vi "Dashboard Main.vi"() -> ()   [LabVIEW 2016]
uses:
  <vilib>/Utility/miscctls.llb/LVRowAndColumnTypeDef.ctl
  <vilib>/event_ctls.llb/eventvkey.ctl
  <vilib>/Rock Robotics/Network Tables/NT Read Numeric Array.vi
  <vilib>/Rock Robotics/WPI/Dashboard/WPI_DashboardLogging Global.vi
panel:
  in  "LED Color":T1={"Hue"={107.81818389892578, 139.81818389892578}, "Sat"={176.07142857142858, 255.0}, "Val"={40.53571428571429, 255.0}} {"Hue" scale=0.0..255.0 scale format="%#_3g"}
  in  "Camera Settings Right":T2={"Frame Rate"=30, "Compression"=30, "Size"=1, "DB Camera Config"=FALSE} {"Frame Rate" scale=1.0..30.0; "Compression" scale=100.0..-1.0; "Size" items=["640x480", "320x240", "160x120"]}
  in  "Camera Name Right":string(combo)="No Camera Selection"
  out "Camera Info":cluster{"Mbps LED":bool, "Mbps":dbl, "fps":dbl} {"fps" format="%#.1g"; "Mbps" format="%#.1g"}
  in  "Camera Settings":T2={"Frame Rate"=30, "Compression"=30, "Size"=1, "DB Camera Config"=FALSE} {"Frame Rate" scale=1.0..30.0; "Compression" scale=100.0..-1.0; "Size" items=["640x480", "320x240", "160x120"]}
  in  "TCP":refnum<k5>
  in  "Rec Mode":enum32{"Stop", "Record", "Playback"}(radio)
  out "Robot IP":string
  out "Image Message":string="Timeout in Camera Communications"
  in  "Dashboard Tab":T3(tab)
  in  "Select Auto":string(combo)="Select Autonomous ..."
  out "NT Connection":bool
  out "Mode":T4(ring)=enum."Auto Disabled"
  out "Camera Image Right":T5(plugin-control)
  in  "DB/String 9":string
  in  "DB/String 8":string
  in  "DB/String 7":string
  in  "DB/String 6":string
  in  "DB/String 5":string
  in  "DB/String 4":string
  in  "DB/String 3":string
  in  "DB/String 2":string
  in  "DB/String 1":string
  in  "DB/String 0":string
  in  "DB/Slider 0":dbl(slide) scale=0.0..5.0
  in  "DB/Slider 1":dbl(slide) scale=0.0..5.0
  in  "DB/Slider 2":dbl(slide) scale=0.0..5.0
  in  "DB/Slider 3":dbl(slide) scale=0.0..5.0
  out "DB/LED 3":bool
  out "DB/LED 2":bool
  out "DB/LED 1":bool
  out "DB/LED 0":bool
  in  "DB/Button 3":bool
  in  "DB/Button 2":bool
  in  "DB/Button 1":bool
  in  "DB/Button 0":bool caption="New Name"
  in  "Test Slider":dbl(slide) scale=0.0..100.0 scale format="%#_3g"
  in  "On/Off":bool caption="Solenoid"
  in  "Test Name":u16(ring) items=["Select the test to run..."]
  in  "Test Tree":string(tree)
  in  "Motor":cluster{"Value":dbl, "Enable":bool} {"Value" scale=-1.0..1.0 scale format="%#_3g"}
  out "Progress":T6 {"Test Progress" scale=0.0..100.0}
  in  "Rev/Fwd":cluster{"Forward":bool, "Reverse":bool}
  in  "Test Ring":u16(ring) items=["Monochrome", "Color"]
  out "Cmd Status":string
  in  "Execute Command":bool
  in  "Command Params":string[][](table)
  in  "Command Selection":i32(listbox)
  in  "CheckList":i32(listbox)
  out "Tree":string(tree)
  out "Camera Image":T5(plugin-control)
  out "Background":bool
  in  "Camera Name":string(combo)="No Camera Selection"
  # "HW"
  # "HW"
  # "This tab is a great place for autonomous settings and robot-specific values.\nPlace controls and indicators inside this tab and match name to\nDashboard Variables on robot. You can also delete this comment."
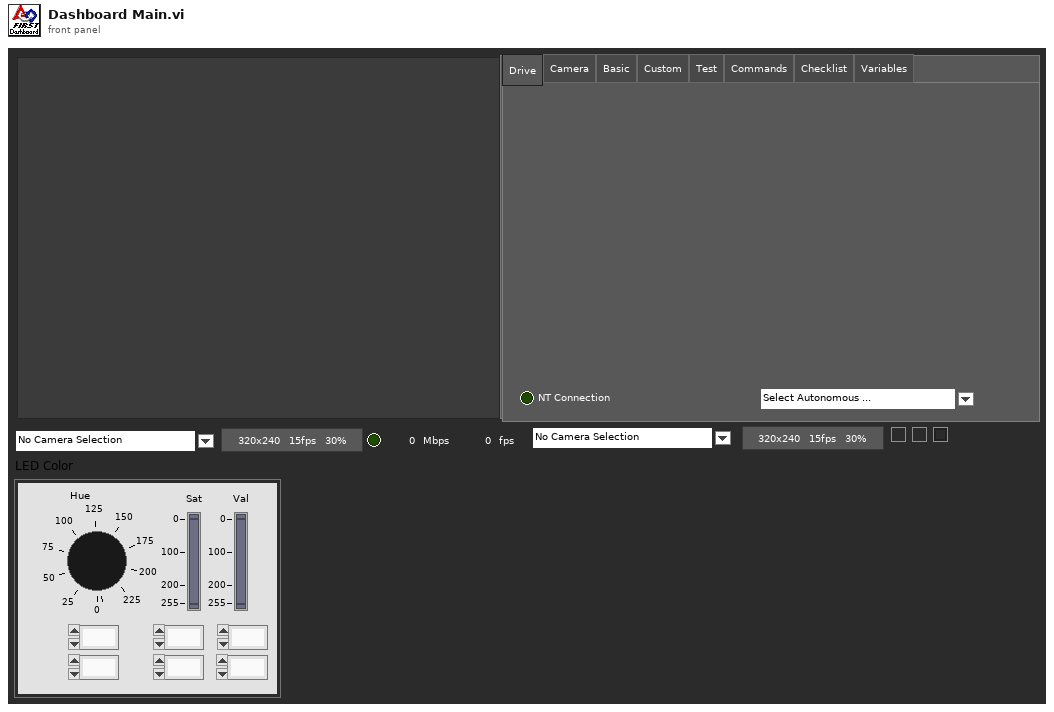
[diagram p1: front panel]
types:
  T1 = cluster{"Hue":cluster{dbl, dbl}, "Sat":cluster{dbl, dbl}, "Val":cluster{dbl, dbl}}
  T2 = cluster{"Frame Rate":i32, "Compression":i32, "Size":u16, "DB Camera Config":bool}
  T3 = enum32{"Drive", "Camera", "Basic", "Custom", "Test", "Commands", "Checklist", "Variables"}
  T4 = enum8{"Tele-Op Disabled", "Tele-Op Enabled", "Auto Disabled", "Auto Enabled", "Test Disabled", "Test Enabled", "Disconnected", "No Code", "E-Stop"}
  T5 = typedef "IMAQ Image.ctl" = refnum<image>
  T6 = cluster{"Test Progress":u8, "Test Progress Text":string}
  T7 = typedef "Image Type" = u32
  T8 = cluster{"IDs":cluster{"RPC field ID":u16, "Unique ID":u16}, "String":string}
  T9 = enum32{"Drive", "Basic", "Custom", "Test", "Checklist", "Variables"}
  T10 = cluster{"Error Strings":string, "Disable Counts":cluster{u16, u16}, "Rail Faults":cluster{u16, u16, u16}, "Robot IP":string, "DB Mode":u8, "Event Info":cluster{"Name":string, "Type":u8, "Number":u16, "Replay":u8}}
  T11 = cluster{"Storage":cluster{"Disk Free":u64, "RAM Block":u32, "RAM free":u32}, "CPU Utilization":cluster{"CPU % ISR":sgl, "CPU % Time Crit":sgl, "CPU % Timed Str":sgl, "CPU % High":sgl, "CPU % Above":sgl, "CPU % Normal":sgl, "CPU % Low":sgl}, "CAN":cluster{"% Bus Utilization":sgl, "Bus Off Cnt":u32, "TX_FIFO Full Cnt":u32, "Receive Error Cnt":u8, "Transmit Error Cnt":u8}, "HID":cluster{"HID Outputs":u32, "Rumble Low":u16, "Rumble High":u16}[]}
  T12 = cluster{"Status bits":cluster{"Test Mode":bool, "Autonomous":bool, "Enabled":bool, "Code Start":bool, "Brownout":bool, "Reserved 2":bool, "Reserved 3":bool, "E-Stop":bool}, "Code Trace":cluster{"Disabled":bool, "TeleOp":bool, "Auto":bool, "Test":bool}, "Controller Type":enum16{"unknown", "cRIO", "roboRio"}, "Code?":enum16{"unknown", "noCode", "code"}, "Battery V":dbl}
  T13 = cluster{"Control Bits":cluster{"TestMode":bool, "Autonomous":bool, "Enabled":bool, "FMS Present":bool, bool, bool, bool, "E-Stop":bool}, "Team Station ":u8, "Countdown":sgl, "Joystick Values":cluster{"Axes":dbl[], "Buttons":bool[], "POVs":i16[]}[]}
  T14 = cluster{"Axes":dbl[], "Buttons":bool[], "POVs":i16[]}[]
  T15 = cluster{"Axes":dbl[], "Buttons":bool[], "POVs":i16[]}
  T16 = cluster{"Camera Image":refnum<vi>, "Dashboard Tab":refnum<vi>, "Background":refnum<vi>, "Rec Mode":refnum<vi>, "Test Slider":refnum<vi>, "On/Off ":refnum<vi>, "Test Ring":refnum<vi>, "Rev/Fwd":refnum<vi>, "Test Name":refnum<vi>, "Motor":refnum<vi>, "Progress":refnum<vi>, "CheckList":refnum<vi>, "Tree":refnum<vi>, "Test Tree":refnum<vi>, "Command Params":refnum<vi>, "Command Selection":refnum<vi>, "Execute Command":refnum<vi>, "Cmd Status":refnum<vi>, "Camera Settings":refnum<vi>, "Camera Name":refnum<vi>, "Camera Info":refnum<vi>, "Camera Settings Right":refnum<vi>, "Camera Name Right":refnum<vi>, "Camera Image Right":refnum<vi>}
  T17 = cluster{"Operation":enum16{"Update", "Clear"}, "Color Box":u32}[]
  T18 = typedef "eventvkey.ctl" = enum16{"ASCII", "Enter", "Return", "Shift", "Ctrl", "Alt", "Cmd", "Opt", "Caps", "NumLock", "Clear", "Break", "Up", "Down", "Left", "Right", "Insert", "Delete", "Home", "End", "PageUp", "PageDown", "Escape", "Help", "Pause", "ScrollLock", "F1", "F2", "F3", "F4", "F5", "F6", "F7", "F8", "F9", "F10", "F11", "F12", "F13", "F14", "F15", "F16", "F17", "F18", "F19", "F20", "F21", "F22", "F23", "F24", "Play", "VolumeUp", "VolumeDown", "Mute", "Two Byte Char"}
  T19 = cluster{"Image Size":bool, "Image Type":bool, "Pixel Value":bool, "ROI Information":bool, "Zoom Factor":bool}
  T20 = cluster{"Operation":enum16{"Update", "Clear"}, "Color Box":u32}
  T21 = typedef "LVRowAndColumnTypeDef.ctl" = cluster{"Row":i32, "Column":i32}
  T22 = cluster{"Shift":bool, "Ctrl":bool, "Alt":bool, "Cmd":bool, "Opt":bool}
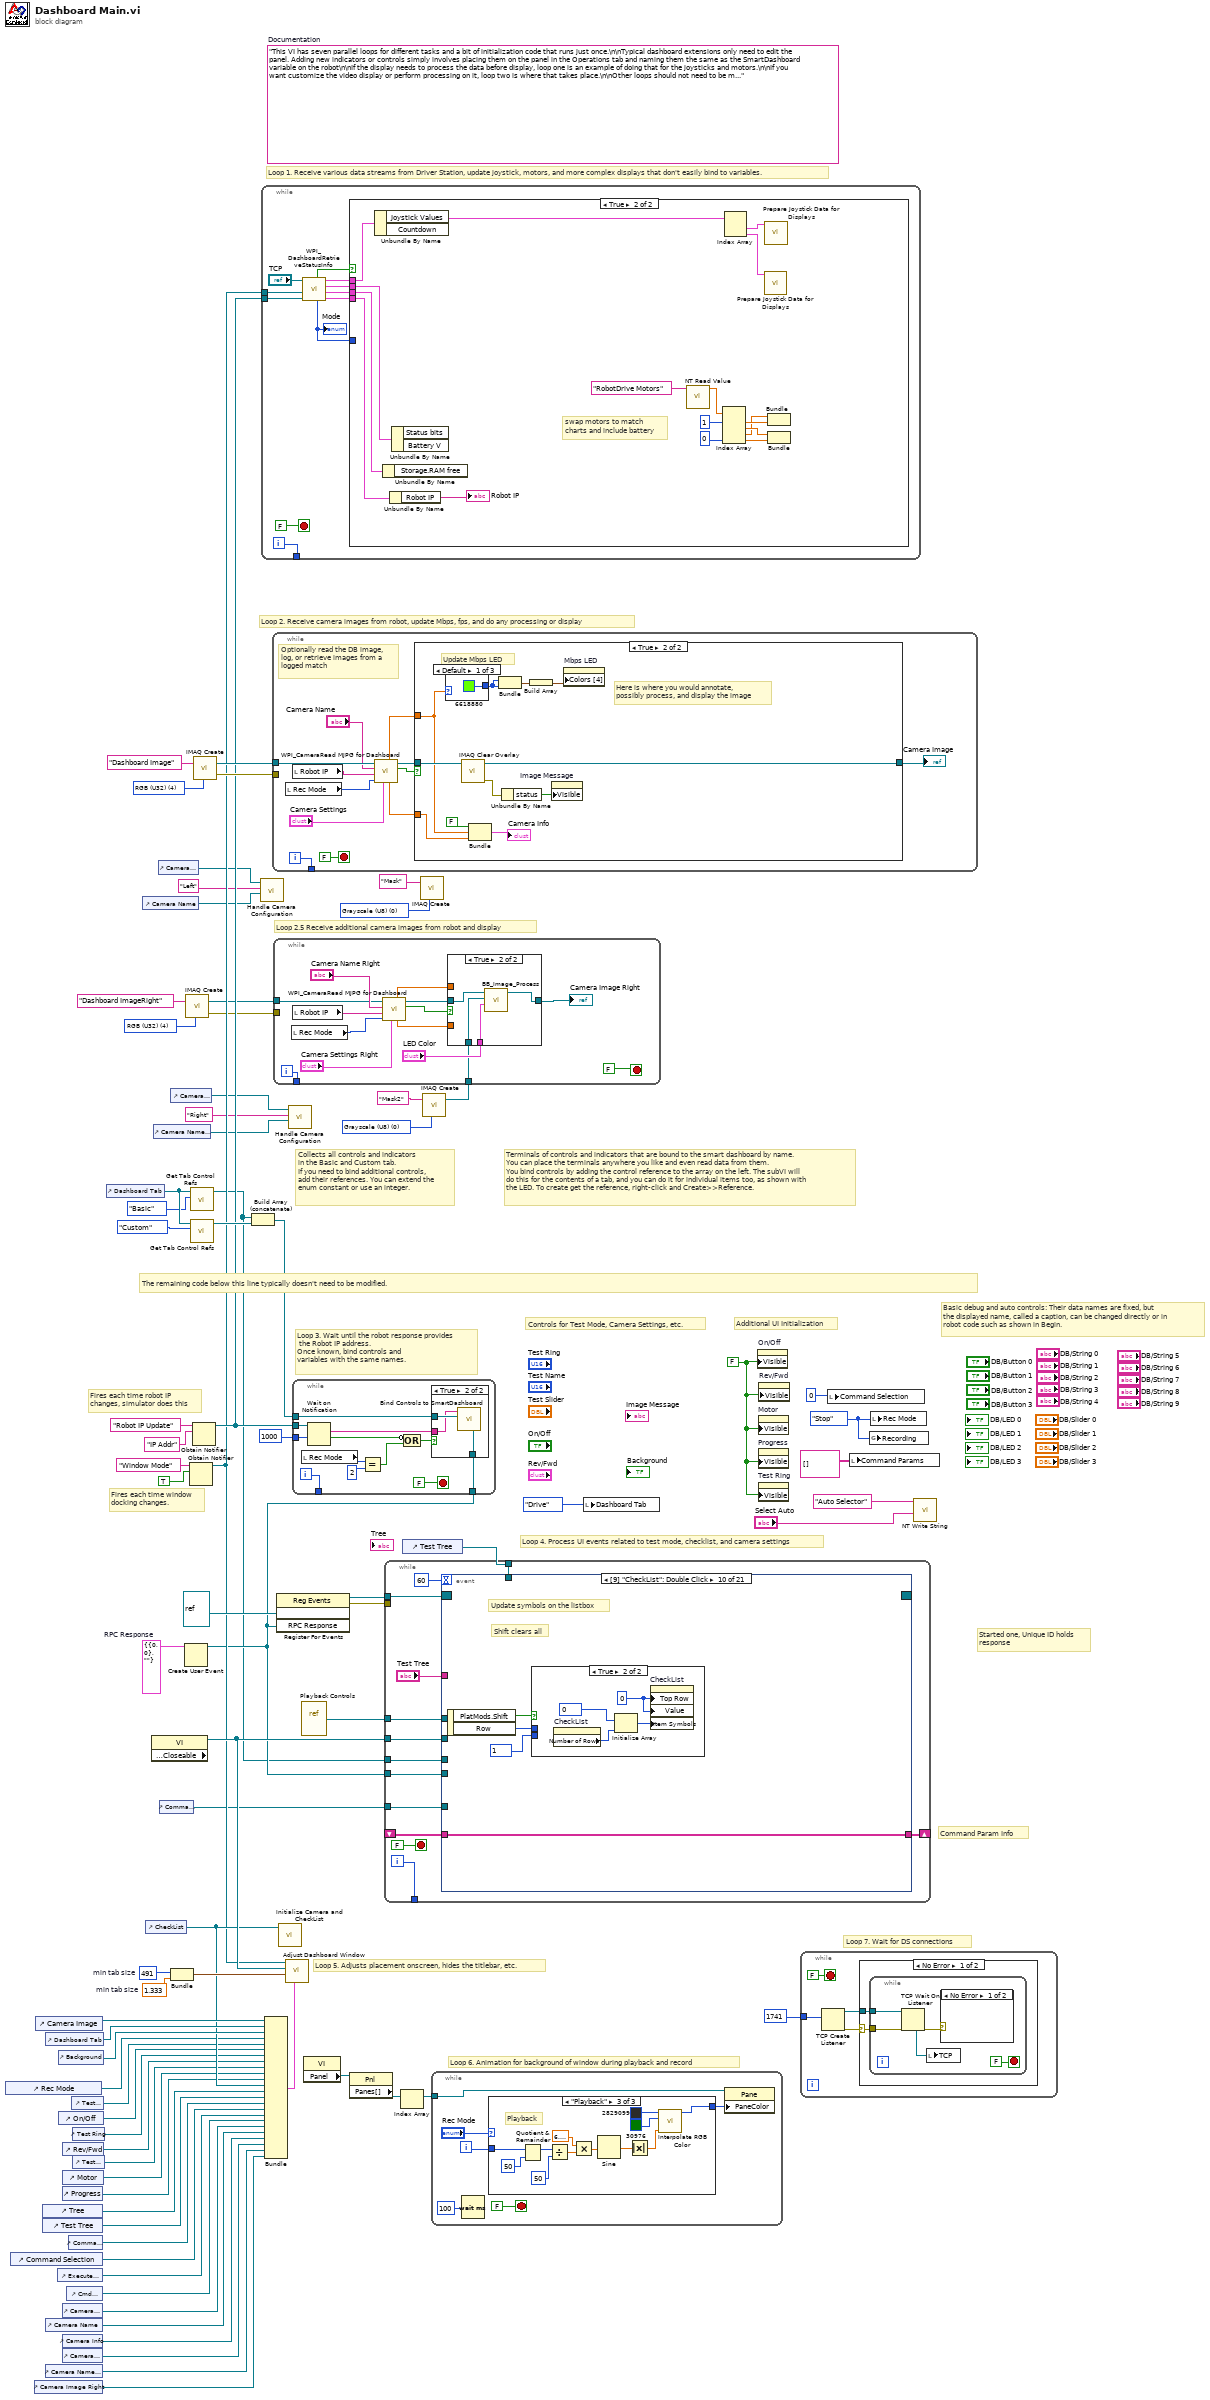
[diagram p0: block diagram]
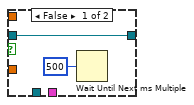
[diagram p2: hidden frame]
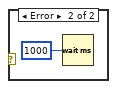
[diagram p3: hidden frame]
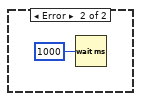
[diagram p4: hidden frame]
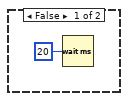
[diagram p5: hidden frame]
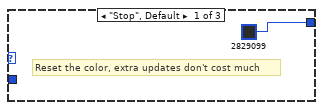
[diagram p6: hidden frame]
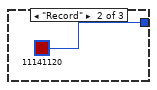
[diagram p7: hidden frame]
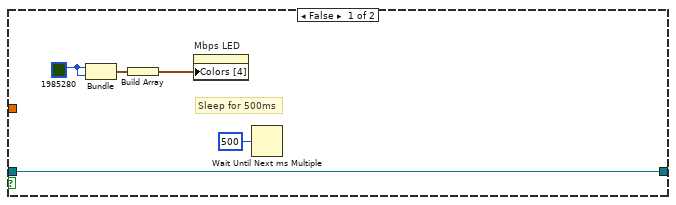
[diagram p9: hidden frame]
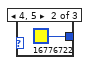
[diagram p10: hidden frame]
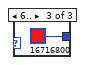
[diagram p11: hidden frame]
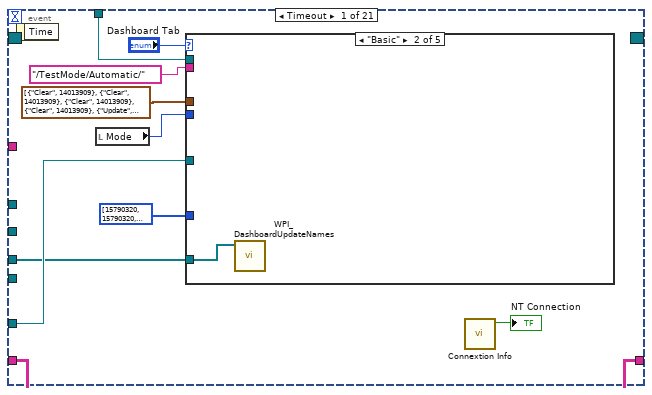
[diagram p12: hidden frame]
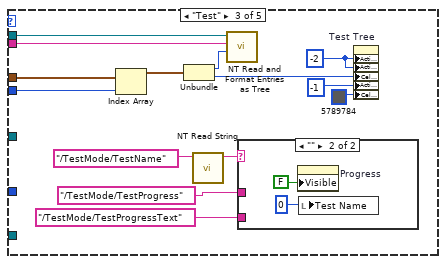
[diagram p14: hidden frame]
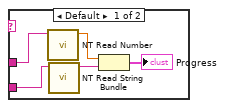
[diagram p15: hidden frame]
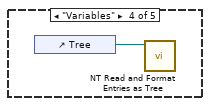
[diagram p16: hidden frame]
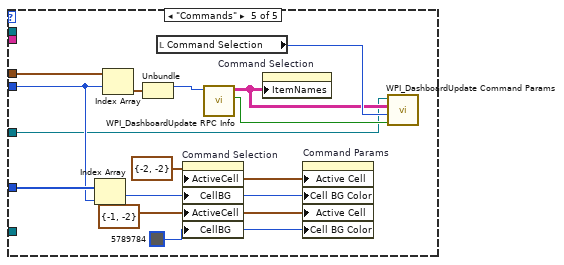
[diagram p17: hidden frame]
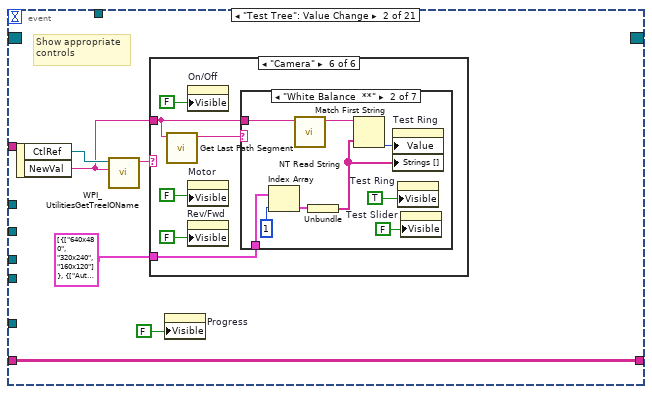
[diagram p18: hidden frame]
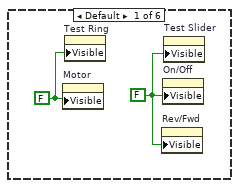
[diagram p19: hidden frame]
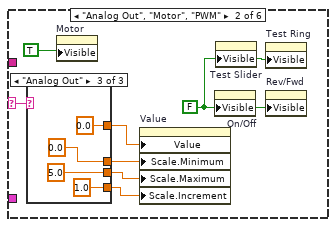
[diagram p20: hidden frame]
diagram:
  w3 = T7 0 items=["Grayscale (U8)", "Grayscale (I16)", "Grayscale (SGL)", "Complex (CSG)", "RGB (U32)", "HSL (U32)", "RGB (U64)", "Grayscale (U16)"] ("Image Type")
  w5 = T7 0 items=["Grayscale (U8)", "Grayscale (I16)", "Grayscale (SGL)", "Complex (CSG)", "RGB (U32)", "HSL (U32)", "RGB (U64)", "Grayscale (U16)"] ("Image Type")
  w15 = T7 4 items=["Grayscale (U8)", "Grayscale (I16)", "Grayscale (SGL)", "Complex (CSG)", "RGB (U32)", "HSL (U32)", "RGB (U64)"] ("Image Type")
  w31 = T8 {"IDs"={"RPC field ID"=0, "Unique ID"=0}, "String"=""}  # RPC Response
  w56 = 491  # min tab size
  w55 = 1.333  # min tab size
  w63 = enum32{"Stop", "Record", "Playback"}."Stop" ("Rec Mode")
  w38 = FALSE ("Visible")
  (unwired) "This VI has seven parallel loops for different tasks and a bit of initialization code that runs just once.\n\nTypical dashboard extensions only need to edit the panel. Adding new indicators or controls simply involves placing them on the panel in the Operations tab and naming them the same as the SmartDashboard variable on the robot\n\nIf the display needs to process the data before display, loop one is an example of doing that for the joysticks and motors.\n\nIf you want customize the video display or perform processing on it, loop two is where that takes place.\n\nOther loops should not need to be modified. They are pretty standard, and document the task they perform."  # Documentation
  w80 = T7 4 items=["Grayscale (U8)", "Grayscale (I16)", "Grayscale (SGL)", "Complex (CSG)", "RGB (U32)", "HSL (U32)", "RGB (U64)"] ("Image Type")
  # "Loop 2.5 Receive additional camera images from robot and display"
  # "Command Param Info"
  # "Started one, Unique ID holds\nresponse"
  # "Loop 7. Wait for DS connections"
  # "Basic debug and auto controls: Their data names are fixed, but\nthe displayed name, called a caption, can be changed directly or in\nrobot code such as shown in Begin."
  # "Controls for Test Mode, Camera Settings, etc."
  # "Additional UI Initialization"
  # "Loop 6. Animation for background of window during playback and record"
  # "Fires each time robot IP\nchanges, simulator does this"
  # "Fires each time window\ndocking changes."
  # "Collects all controls and indicators\nin the Basic and Custom tab.\nIf you need to bind additional controls,\nadd their references. You can extend the\nenum constant or use an integer."
  # "The remaining code below this line typically doesn't need to be modified."
  # "Loop 4. Process UI events related to test mode, checklist, and camera settings"
  # "Terminals of controls and indicators that are bound to the smart dashboard by name.\nYou can place the terminals anywhere you like and even read data from them.\nYou bind controls by adding the control reference to the array on the left. The subVI will\ndo this for the contents of a tab, and you can do it for individual items too, as shown with\nthe LED. To create get the reference, right-click and Create>>Reference."
  # "Loop 3. Wait until the robot response provides\n the Robot IP address.\nOnce known, bind controls and\nvariables with the same names."
  # "Loop 5. Adjusts placement onscreen, hides the titlebar, etc."
  # "Loop 1. Receive various data streams from Driver Station, update joystick, motors, and more complex displays that don't easily bind to variables."
  # "Loop 2. Receive camera images from robot, update Mbps, fps, and do any processing or display"
  n1 = control-ref of="Rec Mode"() -> (w44:refnum<vi>)
  n2 = control-ref of="Command Selection"() -> (w30:refnum<vi>)
  n3 = control-ref of="Camera Image Right"() -> (w6:refnum<vi>)
  n4 = control-ref of="Camera Image"() -> (w58:refnum<vi>)
  n5 = control-ref of="Tree"() -> (w48:refnum<vi>)
  n6 = control-ref of="Test Tree"() -> (w47:refnum<vi>)
  n7 = control-ref of="Dashboard Tab"() -> (w57:refnum<vi>)
  n8 = control-ref of="Camera Name"() -> (w21:refnum<vi>)
  n9 = control-ref of="Camera Name Right"() -> (w7:refnum<vi>)
  n10 = control-ref of="Execute Command"() -> (w32:refnum<vi>)
  n11 = control-ref of="Background"() -> (w53:refnum<vi>)
  n12 = control-ref of="On/Off"() -> (w42:refnum<vi>)
  n13 = control-ref of="Progress"() -> (w39:refnum<vi>)
  n14 = control-ref of="Camera Settings"() -> (w22:refnum<vi>)
  n15 = control-ref of="Camera Info"() -> (w20:refnum<vi>)
  n16 = control-ref of="Camera Settings Right"() -> (w8:refnum<vi>)
  n17 = control-ref of="Rev/Fwd"() -> (w40:refnum<vi>)
  n18 = control-ref of="Motor"() -> (w45:refnum<vi>)
  n19 = control-ref of="Cmd Status"() -> (w26:refnum<vi>)
  n20 = control-ref of="Command Params"() -> (w33:refnum<vi>)
  n21 = control-ref of="Test Slider"() -> (w43:refnum<vi>)
  n22 = control-ref of="Test Ring"() -> (w41:refnum<vi>)
  n23 = control-ref of="Test Name"() -> (w46:refnum<vi>)
  n24 = control-ref of="Dashboard Tab"() -> (w61:refnum<vi>)
  n25 = control-ref of="Camera Name"() -> (w23:refnum<vi>)
  n26 = control-ref of="CheckList"() -> (w49:refnum<vi>)
  n27 = property class="VI" props=["Front Panel.Closeable"]() -> (reference out=w62:refnum<vi>)  [unwired: 2 in, 2 out]
  n28 = control-ref of="Camera Name Right"() -> (w11:refnum<vi>)
  n29 = control-ref of="Camera Settings"() -> (w24:refnum<vi>)
  n30 = control-ref of="Command Params"() -> (w25:refnum<vi>)
  n31 = control-ref of="Camera Settings Right"() -> (w12:refnum<vi>)
  n32 = Bundle("min tab size"=w56, "min tab size"=w55) -> (w54:cluster{"min tab size":i32, "min tab size":dbl})  [unwired: 1 in]
  n33 = Create User Event(user event datatype=w31) -> (user event=w27:refnum<user-event>)  [unwired: 1 in, 1 out]
  n34 = call "IMAQ Create"("Image Name"="Dashboard ImageRight", "Image Type"=w15) -> ("New Image"=w14:T5, "error out"=w13:errorcluster)  [unwired: 2 in, 1 out]
  n35 = Obtain Notifier(name (unnamed)="Window Mode", notification data type=TRUE) -> (notifier out=w36:refnum<notifier>)  [unwired: 2 in, 2 out]
  n36 = call <vilib>:"Get Tab Control Refs.vi"("Page Index"=T9."Basic" ("Dashboard Tab"), "TabControl in"=w61) -> ("ControlsOnPage"=w19:refnum<vi>[])  [unwired: 9 in]
  n37 = call <vilib>:"Get Tab Control Refs.vi"("Page Index"=T9."Custom" ("Dashboard Tab"), "TabControl in"=w61) -> ("ControlsOnPage"=w60:refnum<vi>[])  [unwired: 9 in]
  n38 = Obtain Notifier(name (unnamed)="Robot IP Update", notification data type="IP Addr" ("name (unnamed)")) -> (notifier out=w37:refnum<notifier>)  [unwired: 2 in, 2 out]
  n39 = call "IMAQ Create"("Image Name"="Dashboard Image", "Image Type"=w80) -> ("New Image"=w78:T5, "error out"=w77:errorcluster)  [unwired: 2 in, 1 out]
  n40 = Build Array (concatenate)(w19, w60) -> (w59:refnum<vi>[])
  n41 = call "Handle Camera Configuration.vi"("CameraNameRef"=w23, "Camera File Name"="Left", "ClusterRef"=w24) -> ()  [unwired: 9 in]
  n42 = while {
    tunnel: [w90] -> _
    tunnel: w37 -> [w84]
    tunnel: w36 -> [w81]
    i -> [w90]
    stop <- FALSE stop-if-true
    n43 = call <vilib>:"WPI_DashboardRetrieveStatusInfo.vi"("Binding Refnum"=w84, "Window Mode Notifier"=w81, "TCP Cnx"="TCP") -> ("Power and Errors"=w85:T10, "Robot Metrics"=w88:T11, "Status Info"=w89:T12, "Control Info"=w86:T13, "Robot Mode"=w83:T4, "Process?"=w87:bool)  [unwired: 3 in]
    "Mode" <- w83
    n44 = case shown="True" w87 {
      tunnel: w89 -> [_ w108]
      tunnel: w88 -> [_ w107]
      tunnel: w86 -> [_ w106]
      tunnel: w85 -> [_ w105]
      tunnel: w83 -> [_ _]
      frame False {
        n45 = Wait (ms)(milliseconds to wait=u32 20) -> ()  [unwired: 1 out]
      }
      frame True {
        # "swap motors to match\ncharts and include battery"
        n46 = Unbundle By Name(w106) -> ("Joystick Values"=w98:T14)  [unwired: 1 out]
        n47 = Unbundle By Name(w107) -> ()  [unwired: 1 out]
        n48 = Unbundle By Name(w105) -> ("Robot IP"=→"Robot IP":string)
        n49 = Unbundle By Name(w108) -> ()  [unwired: 2 out]
        n50 = call-poly <vilib>:"NT Read Value.vi"("Name"="RobotDrive Motors") -> ("Numeric Array"=w94:dbl[])  [unwired: 9 in, 1 out]
        n51 = Index Array(array=w94, index #1=1, index #4=0) -> (element #1=w100:dbl, element #2=w101:dbl, element #3=w99:dbl, element #4=w104:dbl)  [unwired: 2 in]
        n52 = Index Array(array=w98) -> (element #1=w97:T15, element #2=w96:T15)  [unwired: 2 in]
        n53 = call "Prepare Joystick Data for Displays.vi"("Joystick Values"=w96) -> ()  [unwired: 8 in, 3 out]
        n54 = call "Prepare Joystick Data for Displays.vi"("Joystick Values"=w97) -> ()  [unwired: 8 in, 3 out]
        n55 = Bundle("Numeric"=w99, "Numeric"=w100) -> ()  [unwired: 1 in, 1 out]
        n56 = Bundle("Numeric"=w101, "Numeric"=w104) -> ()  [unwired: 1 in, 1 out]
      }
    }
  }
  n57 = Bundle("Camera Image"=w58, "Dashboard Tab"=w57, "Background"=w53, "Rec Mode"=w44, "Test Slider"=w43, "On/Off"=w42, "Test Ring"=w41, "Rev/Fwd"=w40, "Test Name"=w46, "Motor"=w45, "Progress"=w39, "CheckList"=w49, "Tree"=w48, "Test Tree"=w47, "Command Params"=w33, "Command Selection"=w30, "Execute Command"=w32, "Cmd Status"=w26, "Camera Settings"=w22, "Camera Name"=w21, "Camera Info"=w20, "Camera Settings Right"=w8, "Camera Name Right"=w7, "Camera Image Right"=w6) -> (w50:T16)  [unwired: 1 in]
  n58 = while {
    tunnel: w78 -> [w118]
    tunnel: w77 -> [_]
    tunnel: [w119] -> _
    i -> [w119]
    stop <- FALSE stop-if-true
    # "Optionally read the DB image,\nlog, or retrieve images from a\nlogged match"
    n59 = local read "Rec Mode"() -> (w114:enum32{"Stop", "Record", "Playback"})
    n60 = local read "Robot IP"() -> (w113:string)
    n61 = call <vilib>:"WPI_CameraRead MJPG for Dashboard.vi"("Camera Settings"="Camera Settings", "Rec Mode"=w114, "Robot IP"=w113, "Camera Name"="Camera Name", "Refnum in"=w118) -> ("Active"=w116:bool, "Refnum out"=w117:T5, "FPS"=w115:dbl, "Bandwidth (Mbps)"=w112:dbl)  [unwired: 3 in]
    n62 = case shown="True" w116 {
      tunnel: w117 -> [w121 w132]
      tunnel: w112 -> [_ w129]
      tunnel: w115 -> [_ w130]
      tunnel: [w121 w126] -> w109
      frame False {
        w123 = u32 1985280 ("Color Box")
        # "Sleep for 500ms"
        n63 = Bundle("Color Box"=w123, "Color Box"=w123) -> (w124:cluster{"Color Box":u32, "Color Box":u32})  [unwired: 1 out]
        n64 = Build Array(w124) -> (w122:cluster{"Color Box":u32, "Color Box":u32}[])
        n65 = property on="Mbps LED" class="Bool (strict)"("Colors [4]"=w122) -> ()  [unwired: 2 in, 2 out]
        n66 = Wait Until Next ms Multiple(millisecond multiple=u32 500) -> ()  [unwired: 1 out]
      }
      frame True {
        # "Here is where you would annotate,\npossibly process, and display the image"
        # "Update Mbps LED"
        n67 = case shown="Default" w129 {
          tunnel: [u32 6618880 ("Color Box") u32 16776722 ("Color Box") u32 16716800 ("Color Box")] -> w133
          frame Default {
          }
          frame 4, 5 {
          }
          frame 6.. {
          }
        }
        n68 = call "IMAQ Clear Overlay"("Image"=w132) -> ("error out"=w135:errorcluster, "Image Out"=w126:T5)  [unwired: 2 in, 7 out]
        n69 = Bundle(FALSE, "Bandwidth (Mbps)"=w129, "FPS"=w130) -> (→"Camera Info":cluster{bool, "Bandwidth (Mbps)":dbl, "FPS":dbl})  [unwired: 1 in]
        n70 = Bundle("Color Box"=w133, "Color Box"=w133) -> (w134:cluster{"Color Box":u32, "Color Box":u32})  [unwired: 1 out]
        n71 = Unbundle By Name(w135) -> ("status"=w136:bool)
        n72 = Build Array(w134) -> (w131:cluster{"Color Box":u32, "Color Box":u32}[])
        n73 = property on="Image Message" class="Str"("Visible"=w136) -> ()  [unwired: 2 in, 2 out]
        n74 = property on="Mbps LED" class="Bool (strict)"("Colors [4]"=w131) -> ()  [unwired: 2 in, 2 out]
      }
    }
    "Camera Image" <- w109
  }
  n75 = register-events(refnum<vi> refnum, w27) -> (reference out=w67:refnum<event-registration>, error out=w66:errorcluster)  [unwired: 2 in]
  n76 = call "Initialize Camera and CheckList.vi"("ListBox in"=w49) -> ()  [unwired: 11 in]
  n77 = call "Adjust Dashboard Window.vi"("Sizing Refnums"=w50, "Size Constraints"=w54, "VI"=w62, "WIn Mode"=w36) -> ()  [unwired: 8 in]
  n78 = call "Handle Camera Configuration.vi"("CameraNameRef"=w11, "Camera File Name"="Right", "ClusterRef"=w12) -> ()  [unwired: 9 in]
  n79 = while {
    tunnel: w59 -> [w151]
    tunnel: w37 -> [w149]
    tunnel: [w147] -> _
    tunnel: u32 1000 ("milliseconds to wait") -> [w146]
    tunnel: w27 -> [w140]
    i -> [w147]
    stop <- FALSE stop-if-true
    n80 = local read "Rec Mode"() -> (w142:enum32{"Stop", "Record", "Playback"})
    n81 = Wait on Notification(notifier=w149, timeout in ms (-1)=w146) -> (notification=w148:string, timed out?=w144:bool)  [unwired: 2 in, 2 out]
    n82 = Equal?(x=w142, y=u16 2 ("Rec Mode")) -> (x = y?=w143:bool)
    n83 = Compound Arithmetic op=OR(invert w144, w143) -> (w145:bool)
    n84 = case shown="True" w145 {
      tunnel: w151 -> [_ w154]
      tunnel: w148 -> [_ w153]
      tunnel: w140 -> [_ w152]
      frame False {
      }
      frame True {
        n85 = call <vilib>:"Bind Controls to SmartDashboard.vi"("RPC ref"=w152, "Bound Control Refs"=w154, "Server IP Address"=w153) -> ()  [unwired: 9 in]
      }
    }
  }
  n86 = vi-ref "Playback Controls.vi"() -> (w68:refnum<vi>)
  n87 = property class="VI"() -> ("Panel"=w70:refnum<vi>)  [unwired: 2 in, 2 out]
  n88 = property class="Pnl"(reference=w70) -> ("Panes[]"=w71:refnum<vi>[])  [unwired: 1 in, 2 out]
  n89 = Index Array(array=w71) -> (element=w69:refnum<vi>)  [unwired: 1 in]
  n90 = control-ref of="Test Tree"() -> (w72:refnum<vi>)
  n91 = while {
    tunnel: [w164] -> _
    tunnel: w72 -> [w163]
    tunnel: w68 -> [w162]
    tunnel: w67 -> [w161]
    tunnel: w66 -> [_]
    tunnel: w62 -> [w160]
    tunnel: w27 -> [w159]
    tunnel: w25 -> [w158]
    shift-right: [w157] -> _
    shift-left: _ -> [w156]
    tunnel: w19 -> [w155]
    i -> [w164]
    stop <- FALSE stop-if-true
    n92 = event shown="[9] \"CheckList\": Double Click" {
      selector: w161 -> [_ _ _ _ _ _ _ _ _ _ _ _ _ _ _ _ _ _ _ _ _]
      dyn-events: [_ _ _ _ _ _ _ _ _ _ _ _ _ _ _ _ w420 _ _ _ _] -> _
      timeout: u32 60 ("milliseconds to wait") -> [_ _ _ _ _ _ _ _ _ _ _ _ _ _ _ _ _ _ _ _ _]
      tunnel: w163 -> [w176 _ _ _ _ _ _ _ _ _ _ _ _ _ _ _ _ _ _ _ _]
      tunnel: "Test Tree" -> [_ _ _ _ _ _ _ _ _ _ _ w387 w395 w397 w401 w409 _ _ _ _ _]
      tunnel: w162 -> [_ _ _ _ _ _ _ _ _ _ _ _ _ _ _ _ w422 _ w440 _ _]
      tunnel: w160 -> [_ _ _ _ _ _ _ _ _ _ _ _ _ _ _ _ w418 _ _ _ _]
      tunnel: w159 -> [_ _ _ _ _ _ _ _ _ _ _ _ _ _ _ _ w414 _ _ _ _]
      tunnel: w158 -> [w171 _ _ _ _ _ w338 _ _ _ _ _ _ _ _ _ _ _ _ _ _]
      tunnel: [w170 w215 w317 w322 w331 w335 w336 w345 w355 w362 w374 w386 w393 w396 w400 w408 w413 w435 w437 w441 w452] -> w157
      tunnel: w156 -> [w170 w215 w317 w322 w331 w335 w336 _ _ w362 w374 w386 w393 w396 w400 w408 w413 w435 w437 w441 w452]
      tunnel: w155 -> [w168 _ _ _ _ _ _ _ _ _ _ _ _ _ _ _ _ _ _ _ _]
      event Timeout {
        n93 = event-data() -> ()  [unwired: 1 in, 1 out]
        n94 = local read "Mode"() -> (w173:T4)
        n95 = case shown="\"Basic\"" "Dashboard Tab" {
          tunnel: w176 -> [_ _ w192 _ _]
          tunnel: "/TestMode/Automatic/" ("Name Pattern") -> [_ _ w191 _ _]
          tunnel: T17 [{"Operation"=enum."Clear", "Color Box"=14013909}, {"Operation"=enum."Clear", "Color Box"=14013909}, {"Operation"=enum."Clear", "Color Box"=14013909}, {"Operation"=enum."Clear", "Color Box"=14013909}, {"Operation"=enum."Update", "Color Box"=14013909}, {"Operation"=enum."Update", "Color Box"=16777215}, {"Operation"=enum."Clear", "Color Box"=14013909}, {"Operation"=enum."Clear", "Color Box"=14013909}, {"Operation"=enum."Clear", "Color Box"=14013909}] -> [_ _ w184 _ w208]
          tunnel: w173 -> [_ _ w183 _ w207]
          tunnel: u32[] [15790320, 15790320, 15790320, 15790320, 16777215, 16777215, 15790320, 15790320, 15790320] -> [_ _ _ _ w213]
          tunnel: w171 -> [_ _ _ _ w201]
          tunnel: w168 -> [_ w178 _ _ _]
          frame "Custom", Default {
          }
          frame "Basic" {
            n96 = call <vilib>:"WPI_DashboardUpdateNames.vi"("Controls on Tab"=w178) -> ()  [unwired: 11 in]
          }
          frame "Test" {
            w190 = -2 ("Active Item:Row Number")
            n97 = Index Array(array=w184, index=w183) -> (element=w185:T20)
            n98 = Unbundle(w185) -> ("Operation"=w186:enum16{"Update", "Clear"}, "Color Box"=w187:u32)
            n99 = call <vilib>:"NT Read String.vi"("Name"="/TestMode/TestName") -> ("String"=w181:string)  [unwired: 9 in, 1 out]
            n100 = call <vilib>:"NT Read and Format Entries as Tree.vi"("Operation"=w186, "Name Pattern"=w191, "Tree Refnum"=w192) -> ()  [unwired: 7 in, 2 out]
            n101 = case shown="\"\"" w181 {
              tunnel: "/TestMode/TestProgress" ("Name") -> [w194 _]
              tunnel: "/TestMode/TestProgressText" ("Name") -> [w193 _]
              frame Default {
                n102 = call <vilib>:"NT Read Number.vi"("Name"=w194) -> ("Numeric"=w195:dbl)  [unwired: 9 in, 1 out]
                n103 = call <vilib>:"NT Read String.vi"("Name"=w193) -> ("String"=w196:string)  [unwired: 9 in, 1 out]
                n104 = Bundle("Numeric"=w195, "String"=w196) -> (→"Progress":cluster{"Numeric":dbl, "String":string})  [unwired: 1 in]
              }
              frame "" {
                n105 = property on="Progress" class="Clust (strict)"("Visible"=FALSE) -> ()  [unwired: 2 in, 2 out]
                n106 = local write "Test Name"(u16 0) -> ()
              }
            }
            n107 = property on="Test Tree" class="Tree (strict)"("Active Item Row Number"=w190, "ActiveColNum"=w190, "CellBG"=w187, "Active Item Row Number"=-1 ("Active Item:Row Number"), "CellBG"=u32 5789784 ("Color Box")) -> ()  [unwired: 2 in, 2 out]
          }
          frame "Variables" {
            n108 = control-ref of="Tree"() -> (w200:refnum<vi>)
            n109 = call <vilib>:"NT Read and Format Entries as Tree.vi"("Tree Refnum"=w200) -> ()  [unwired: 9 in, 2 out]
          }
          frame "Commands" {
            w209 = u32 5789784 ("Color Box")
            w210 = T21 {"Row"=-1, "Column"=-2} ("Active Cell:Active Cell")
            w212 = T21 {"Row"=-2, "Column"=-2} ("Active Cell:Active Cell")
            n110 = Index Array(array=w213, index=w207) -> (element=w211:u32)
            n111 = Index Array(array=w208, index=w207) -> (element=w206:T20)
            n112 = Unbundle(w206) -> ("Operation"=w205:enum16{"Update", "Clear"})  [unwired: 1 out]
            n113 = local read "Command Selection"() -> (w204:i32)
            n114 = property on="Command Selection" class="MCListbox (strict)"("ActiveCell"=w212, "CellBG"=w211, "ActiveCell"=w210, "CellBG"=w209) -> ()  [unwired: 2 in, 2 out]
            n115 = call <vilib>:"WPI_DashboardUpdate RPC Info.vi"("Operation"=w205) -> ("update"=w203:bool, "commands"=w202:string[][])  [unwired: 9 in]
            n116 = property on="Command Selection" class="MCListbox (strict)"("ItemNames"=w202) -> ()  [unwired: 2 in, 2 out]
            n117 = property on="Command Params" class="Tbl (strict)"("Active Cell"=w212, "Cell BG Color"=w211, "Active Cell"=w210, "Cell BG Color"=w209) -> ()  [unwired: 2 in, 2 out]
            n118 = call <vilib>:"WPI_DashboardUpdate Command Params.vi"("Update"=w203, "NewVal"=w204, "Commands"=w202, "Param Tbl"=w201) -> ()  [unwired: 7 in, 1 out]
          }
        }
        n119 = call <vilib>:"Connextion Info.vi"() -> ("Connected"=→"NT Connection":bool)  [unwired: 10 in, 1 out]
      }
      event "Test Tree": Value Change {
        # "Show appropriate\ncontrols"
        n120 = event-data() -> ("CtlRef"=w218:refnum<vi>, "NewVal"=w216:string)  [unwired: 1 in]
        n121 = call <vilib>:"WPI_UtilitiesGetTreeIOName.vi"("NewVal"=w216, "TreeControl in"=w218) -> ("I/O Name"=w219:string)  [unwired: 9 in]
        n122 = case shown="\"Camera\"" w219 {
          selector: w219 -> [_ w226 _ w248 w257 _]
          tunnel: w216 -> [_ _ w245 w247 _ w264]
          tunnel: cluster{string[]}[] [{["640x480", "320x240", "160x120"]}, {["Auto", "Fixed indoor", "Fixed outdoor 1", "Fixed outdoor 2", "Fixed fluorescent 1", "Fixed fluorescent 2", "Hold current"]}, {["Auto", "Flicker-free 50 Hz", "Flicker-free 60 Hz", "Hold current"]}, {["None", "Prioritize frame rate", "Prioritize image quality"]}, {["Monochrome", "Color"]}] -> [_ _ _ _ _ w263]
          frame Default {
            w221 = FALSE ("Visible")
            w220 = FALSE ("Visible")
            n123 = property on="Motor" class="Clust (strict)"("Visible"=w220) -> ()  [unwired: 2 in, 2 out]
            n124 = property on="Test Ring" class="Ring (strict)"("Visible"=w220) -> ()  [unwired: 2 in, 2 out]
            n125 = property on="Rev/Fwd" class="Clust (strict)"("Visible"=w221) -> ()  [unwired: 2 in, 2 out]
            n126 = property on="On/Off" class="Bool (strict)"("Visible"=w221) -> ()  [unwired: 2 in, 2 out]
            n127 = property on="Test Slider" class="Slide (strict)"("Visible"=w221) -> ()  [unwired: 2 in, 2 out]
          }
          frame "Analog Out", "Motor", "PWM" {
            w227 = FALSE ("Visible")
            n128 = case shown="\"Analog Out\"" w226 {
              tunnel: [1.0 ("Value") -1.0 ("Value") 0.0 ("Value")] -> w225
              tunnel: [255.0 ("Value") 1.0 ("Value") 5.0 ("Value")] -> w224
              tunnel: [128.0 ("Value") 0.0 ("Value") 0.0 ("Value")] -> w223
              tunnel: [64.0 ("Value") 0.5 ("Value") 1.0 ("Value")] -> w222
              frame "PWM" {
              }
              frame "Motor", Default {
              }
              frame "Analog Out" {
              }
            }
            n129 = property on="Motor" class="Clust (strict)"("Visible"=TRUE) -> ()  [unwired: 2 in, 2 out]
            n130 = property on="Value" class="Slide (strict)"("Value"=w223, "Scale.Minimum"=w225, "Scale.Maximum"=w224, "Scale.Increment"=w222) -> ()  [unwired: 2 in, 2 out]
            n131 = property on="On/Off" class="Bool (strict)"("Visible"=w227) -> ()  [unwired: 2 in, 2 out]
            n132 = property on="Test Slider" class="Slide (strict)"("Visible"=w227) -> ()  [unwired: 2 in, 2 out]
            n133 = property on="Test Ring" class="Ring (strict)"("Visible"=w227) -> ()  [unwired: 2 in, 2 out]
            n134 = property on="Rev/Fwd" class="Clust (strict)"("Visible"=w227) -> ()  [unwired: 2 in, 2 out]
          }
          frame "Servo" {
            w243 = FALSE ("Visible")
            n135 = call <vilib>:"NT Read Number.vi"("Name"=w245) -> ("Numeric"=w244:dbl)  [unwired: 9 in, 1 out]
            n136 = property on="Test Slider" class="Slide (strict)"("Visible"=TRUE, "Scale.Maximum"=170.0 ("Scale.Range:Maximum")) -> ()  [unwired: 2 in, 2 out]
            n137 = local write "Test Slider"(w244) -> ()
            n138 = property on="Motor" class="Clust (strict)"("Visible"=w243) -> ()  [unwired: 2 in, 2 out]
            n139 = property on="Rev/Fwd" class="Clust (strict)"("Visible"=w243) -> ()  [unwired: 2 in, 2 out]
            n140 = property on="On/Off" class="Bool (strict)"("Visible"=w243) -> ()  [unwired: 2 in, 2 out]
            n141 = property on="Test Ring" class="Ring (strict)"("Visible"=w243) -> ()  [unwired: 2 in, 2 out]
          }
          frame "Relay", "Solenoid" {
            w246 = FALSE ("Visible")
            n142 = property on="Motor" class="Clust (strict)"("Visible"=w246) -> ()  [unwired: 2 in, 2 out]
            n143 = property on="Test Slider" class="Slide (strict)"("Visible"=w246) -> ()  [unwired: 2 in, 2 out]
            n144 = Search and Replace String(input string=w247, search string="/Value  **", replace string="/Direction") -> (result string=w253:string)  [unwired: 5 in, 3 out]
            n145 = property on="Test Ring" class="Ring (strict)"("Visible"=w246) -> ()  [unwired: 2 in, 2 out]
            n146 = call <vilib>:"NT Read String.vi"("Name"=w253) -> ("String"=w251:string)  [unwired: 9 in, 1 out]
            n147 = Equal?(x="Both directions", y=w251) -> (x = y?=w249:bool)
            n148 = Not(x=w249) -> (.not. x?=w250:bool)
            n149 = property on="Rev/Fwd" class="Clust (strict)"("Visible"=w249) -> ()  [unwired: 2 in, 2 out]
            n150 = property on="On/Off" class="Bool (strict)"("Visible"=w250, "Caption.Text"=w248) -> ()  [unwired: 2 in, 2 out]
          }
          frame "Compressor", "Digital Out" {
            w256 = FALSE ("Visible")
            # "Get direction and finish"
            n151 = property on="Motor" class="Clust (strict)"("Visible"=w256) -> ()  [unwired: 2 in, 2 out]
            n152 = property on="Test Slider" class="Slide (strict)"("Visible"=w256) -> ()  [unwired: 2 in, 2 out]
            n153 = property on="Test Ring" class="Ring (strict)"("Visible"=w256) -> ()  [unwired: 2 in, 2 out]
            n154 = property on="On/Off" class="Bool (strict)"("Visible"=TRUE, "Caption.Text"=w257) -> ()  [unwired: 2 in, 2 out]
            n155 = property on="Rev/Fwd" class="Clust (strict)"("Visible"=FALSE) -> ()  [unwired: 2 in, 2 out]
          }
          frame "Camera" {
            n156 = call <vilib>:"Get Last Path Segment.vi"("String in"=w264) -> ("String out"=w265:string)  [unwired: 10 in]
            n157 = property on="On/Off" class="Bool (strict)"("Visible"=FALSE) -> ()  [unwired: 2 in, 2 out]
            n158 = property on="Motor" class="Clust (strict)"("Visible"=FALSE) -> ()  [unwired: 2 in, 2 out]
            n159 = property on="Rev/Fwd" class="Clust (strict)"("Visible"=FALSE) -> ()  [unwired: 2 in, 2 out]
            n160 = case shown="\"White Balance  **\"" w265 {
              tunnel: w264 -> [w271 w280 w289 w298 w307 _ w313]
              tunnel: w263 -> [w269 w277 w286 w295 w304 _ _]
              frame "Size  **" {
                n161 = Index Array(array=w269) -> (element=w268:cluster{string[]})  [unwired: 1 in]
                n162 = call <vilib>:"NT Read String.vi"("Name"=w271) -> ("String"=w270:string)  [unwired: 9 in, 1 out]
                n163 = Unbundle(w268) -> (w266:string[])
                n164 = Match First String(2:w266, 3:w270) -> (0:w267:i32)  [unwired: 1 out]
                n165 = property on="Test Ring" class="Ring (strict)"("Value"=w267, "Strings []"=w266) -> ()  [unwired: 2 in, 2 out]
                n166 = property on="Test Ring" class="Ring (strict)"("Visible"=TRUE) -> ()  [unwired: 2 in, 2 out]
                n167 = property on="Test Slider" class="Slide (strict)"("Visible"=FALSE) -> ()  [unwired: 2 in, 2 out]
              }
              frame "White Balance  **" {
                n168 = Index Array(array=w277, index=1) -> (element=w278:cluster{string[]})
                n169 = call <vilib>:"NT Read String.vi"("Name"=w280) -> ("String"=w279:string)  [unwired: 9 in, 1 out]
                n170 = Unbundle(w278) -> (w275:string[])
                n171 = Match First String(2:w275, 3:w279) -> (0:w274:i32)  [unwired: 1 out]
                n172 = property on="Test Ring" class="Ring (strict)"("Value"=w274, "Strings []"=w275) -> ()  [unwired: 2 in, 2 out]
                n173 = property on="Test Ring" class="Ring (strict)"("Visible"=TRUE) -> ()  [unwired: 2 in, 2 out]
                n174 = property on="Test Slider" class="Slide (strict)"("Visible"=FALSE) -> ()  [unwired: 2 in, 2 out]
              }
              frame "Exposure  **" {
                n175 = Index Array(array=w286, index=2) -> (element=w287:cluster{string[]})
                n176 = call <vilib>:"NT Read String.vi"("Name"=w289) -> ("String"=w288:string)  [unwired: 9 in, 1 out]
                n177 = Unbundle(w287) -> (w283:string[])
                n178 = Match First String(2:w283, 3:w288) -> (0:w284:i32)  [unwired: 1 out]
                n179 = property on="Test Ring" class="Ring (strict)"("Value"=w284, "Strings []"=w283) -> ()  [unwired: 2 in, 2 out]
                n180 = property on="Test Ring" class="Ring (strict)"("Visible"=TRUE) -> ()  [unwired: 2 in, 2 out]
                n181 = property on="Test Slider" class="Slide (strict)"("Visible"=FALSE) -> ()  [unwired: 2 in, 2 out]
              }
              frame "Exposure Priority  **" {
                n182 = Index Array(array=w295, index=3) -> (element=w296:cluster{string[]})
                n183 = call <vilib>:"NT Read String.vi"("Name"=w298) -> ("String"=w297:string)  [unwired: 9 in, 1 out]
                n184 = Unbundle(w296) -> (w292:string[])
                n185 = Match First String(2:w292, 3:w297) -> (0:w293:i32)  [unwired: 1 out]
                n186 = property on="Test Ring" class="Ring (strict)"("Value"=w293, "Strings []"=w292) -> ()  [unwired: 2 in, 2 out]
                n187 = property on="Test Ring" class="Ring (strict)"("Visible"=TRUE) -> ()  [unwired: 2 in, 2 out]
                n188 = property on="Test Slider" class="Slide (strict)"("Visible"=FALSE) -> ()  [unwired: 2 in, 2 out]
              }
              frame "Color Enable  **" {
                n189 = Index Array(array=w304, index=4) -> (element=w305:cluster{string[]})
                n190 = call <vilib>:"NT Read String.vi"("Name"=w307) -> ("String"=w306:string)  [unwired: 9 in, 1 out]
                n191 = Unbundle(w305) -> (w301:string[])
                n192 = Match First String(2:w301, 3:w306) -> (0:w302:i32)  [unwired: 1 out]
                n193 = property on="Test Ring" class="Ring (strict)"("Value"=w302, "Strings []"=w301) -> ()  [unwired: 2 in, 2 out]
                n194 = property on="Test Ring" class="Ring (strict)"("Visible"=TRUE) -> ()  [unwired: 2 in, 2 out]
                n195 = property on="Test Slider" class="Slide (strict)"("Visible"=FALSE) -> ()  [unwired: 2 in, 2 out]
              }
              frame Default {
                n196 = property on="Test Ring" class="Ring (strict)"("Visible"=FALSE) -> ()  [unwired: 2 in, 2 out]
                n197 = property on="Test Slider" class="Slide (strict)"("Visible"=FALSE) -> ()  [unwired: 2 in, 2 out]
              }
              frame "Brightness  **", "Color Level  **", "Compression  **", "FPS  **", "Sharpness  **" {
                n198 = call <vilib>:"NT Read Number.vi"("Name"=w313) -> ("Numeric"=w312:dbl)  [unwired: 9 in, 1 out]
                n199 = local write "Test Slider"(w312) -> ()
                n200 = property on="Test Slider" class="Slide (strict)"("Visible"=TRUE, "Scale.Maximum"=100.0 ("Scale.Range:Maximum")) -> ()  [unwired: 2 in, 2 out]
                n201 = property on="Test Ring" class="Ring (strict)"("Visible"=FALSE) -> ()  [unwired: 2 in, 2 out]
              }
            }
          }
        }
        n202 = property on="Progress" class="Clust (strict)"("Visible"=FALSE) -> ()  [unwired: 2 in, 2 out]
      }
      event "Test Name": Mouse Enter {
        # "Populate the ring with the list of tests"
        n203 = event-data() -> ()  [unwired: 1 in, 1 out]
        n204 = call <vilib>:"NT Read String Array.vi"("Name"="/TestMode/TestList") -> ("String Array"=w321:string[])  [unwired: 9 in, 1 out]
        n205 = Build Array (concatenate)("Select the test to run...", w321) -> (w320:string[])
        n206 = property on="Test Name" class="Ring (strict)"("Strings []"=w320) -> ()  [unwired: 2 in, 2 out]
      }
      event "Test Name": Value Change {
        w323 = FALSE ("Visible")
        # "Tell the robot the test name to run"
        n207 = event-data() -> ("NewVal"=w327:u16)  [unwired: 1 in]
        n208 = property on="Test Name" class="Ring (strict)"() -> ("Strings []"=w328:string[])  [unwired: 2 in, 2 out]
        n209 = local write "Progress"(T6 {"Test Progress"=0, "Test Progress Text"=""} ("Progress")) -> ()
        n210 = Index Array(array=w328, index=w327) -> (element=w326:string)
        n211 = call <vilib>:"NT Write String.vi"("String"=w326, "Name"="/TestMode/TestName") -> ()  [unwired: 9 in, 1 out]
        n212 = property on="Progress" class="Clust (strict)"("Visible"=TRUE) -> ()  [unwired: 2 in, 2 out]
        n213 = property on="Motor" class="Clust (strict)"("Visible"=w323) -> ()  [unwired: 2 in, 2 out]
        n214 = property on="Test Slider" class="Slide (strict)"("Visible"=w323) -> ()  [unwired: 2 in, 2 out]
        n215 = property on="On/Off" class="Bool (strict)"("Visible"=w323) -> ()  [unwired: 2 in, 2 out]
        n216 = property on="Rev/Fwd" class="Clust (strict)"("Visible"=w323) -> ()  [unwired: 2 in, 2 out]
        n217 = property on="Test Ring" class="Ring (strict)"("Visible"=w323) -> ()  [unwired: 2 in, 2 out]
      }
      event "Select Auto": Mouse Enter {
        # "Populate the combo box with the list of autonomous options"
        n218 = event-data() -> ()  [unwired: 1 in, 1 out]
        n219 = call <vilib>:"NT Read String Array.vi"("Name"="Auto List") -> ("String Array"=w330:string[])  [unwired: 9 in, 1 out]
        n220 = property on="Select Auto" class="CmbBox"("Strings[]"=w330) -> ()  [unwired: 2 in, 2 out]
      }
      event "Select Auto": Value Change {
        # "User modified the Auto Selection. Write to NT variable so robot knows."
        n221 = event-data() -> ("NewVal"=w333:string)  [unwired: 1 in]
        n222 = call <vilib>:"NT Write String.vi"("String"=w333, "Name"="Auto Selector") -> ()  [unwired: 9 in, 1 out]
      }
      event "Command Selection": Value Change {
        # "Get the params and show in table"
        n223 = event-data() -> ("NewVal"=w339:i32)  [unwired: 1 in]
        n224 = property on="Command Selection" class="MCListbox (strict)"() -> ("ItemNames"=w337:string[][])  [unwired: 2 in, 2 out]
        n225 = call <vilib>:"WPI_DashboardUpdate Command Params.vi"("NewVal"=w339, "Commands"=w337, "Param Tbl"=w338) -> ()  [unwired: 8 in, 1 out]
      }
      event "Execute Command": Value Change {
        # "Started one, Unique ID holds\nresponse"
        n226 = event-data() -> ()  [unwired: 1 in, 1 out]
        n227 = property on="Command Selection" class="MCListbox (strict)"() -> ("ItemNames"=w350:string[][])  [unwired: 2 in, 2 out]
        n228 = Index Array(array=w350, index (row)="Command Selection", index (col)=0) -> (element=w348:string)
        n229 = call <vilib>:"Invoke Commands.vi"("Command Params"="Command Params", "Function Name"=w348) -> ("Params"=w344:u8, "Started"=w343:bool)  [unwired: 7 in, 1 out]
        n230 = Array Subset(array="Command Params", length (row)=w344) -> (w345:string[][])  [unwired: 3 in]
        n231 = Select(t="Executing" ("Cmd Status"), s=w343, f="" ("Cmd Status")) -> (s? t:f=→"Cmd Status":string)
      }
      event "Command Selection": Double Click {
        n232 = event-data() -> ("Row"=w358:i32)  [unwired: 1 in]
        n233 = property on="Command Selection" class="MCListbox (strict)"() -> ("ItemNames"=w361:string[][])  [unwired: 2 in, 2 out]
        n234 = local read "Command Params"() -> (w357:string[][])
        n235 = Index Array(array=w361, index (row)=w358, index (col)=0) -> (element=w359:string)
        n236 = call <vilib>:"Invoke Commands.vi"("Command Params"=w357, "Function Name"=w359) -> ("Params"=w356:u8, "Started"=w351:bool)  [unwired: 7 in, 1 out]
        n237 = Array Subset(array=w357, length (row)=w356) -> (w355:string[][])  [unwired: 3 in]
        n238 = Select(t="Executing" ("Cmd Status"), s=w351, f="" ("Cmd Status")) -> (s? t:f=w352:string)
        n239 = local write "Cmd Status"(w352) -> ()
      }
      event "CheckList": Double Click {
        # "Shift clears all"
        # "Update symbols on the listbox"
        n240 = event-data() -> ("PlatMods.Shift"=w363:bool, "Row"=w365:i32)  [unwired: 1 in]
        n241 = case shown="True" w363 {
          tunnel: w365 -> [w369 _]
          tunnel: 1 -> [w368 _]
          frame False {
            n242 = property on="CheckList" class="LstBox (strict)"() -> ("Item Symbols"=w367:i32[])  [unwired: 2 in, 2 out]
            n243 = Replace Array Subset(array=w367, new element=w368, index=w369) -> (w366:i32[])
            n244 = property on="CheckList" class="LstBox (strict)"("Item Symbols"=w366) -> ()  [unwired: 2 in, 2 out]
          }
          frame True {
            w370 = 0 ("Top Row")
            n245 = property on="CheckList" class="LstBox (strict)"() -> ("Number of Rows"=w372:u32)  [unwired: 2 in, 2 out]
            n246 = Initialize Array(0, w372) -> (w371:i32[])
            n247 = property on="CheckList" class="LstBox (strict)"("Top Row"=w370, "Value"=w370, "Item Symbols"=w371) -> ()  [unwired: 2 in, 2 out]
          }
        }
      }
      event "CheckList": Key Down {
        # "Update symbols on the listbox\nLeft and right keys check and uncheck"
        n248 = event-data() -> ("VKey"=w376:T18)  [unwired: 1 in]
        n249 = case shown="\"Left\", \"Right\"" w376 {
          selector: w376 -> [w381 _]
          tunnel: eventvkey."Left" ("VKey") -> [w379 _]
          frame "Left", "Right" {
            n250 = Equal?(x=w379, y=w381) -> (x = y?=w380:bool)
            n251 = Select(t=0, s=w380, f=1) -> (s? t:f=w382:i32)
            n252 = property on="CheckList" class="LstBox (strict)"() -> ("Item Symbols"=w385:i32[])  [unwired: 2 in, 2 out]
            n253 = Replace Array Subset(array=w385, new element=w382, index="CheckList") -> (w384:i32[])
            n254 = property on="CheckList" class="LstBox (strict)"("Item Symbols"=w384) -> ()  [unwired: 2 in, 2 out]
          }
          frame Default {
          }
        }
      }
      event "Motor.Enable": Value Change {
        # "When the test mode otor enable helper is set, update that\ntree row item's value"
        n255 = event-data() -> ("NewVal"=w391:bool)  [unwired: 1 in]
        n256 = Unbundle("Motor") -> ("Value"=w390:dbl)  [unwired: 1 out]
        n257 = Select(t=w390, s=w391, f=0.0) -> (s? t:f=w388:dbl)
        n258 = call <vilib>:"NT Write Number.vi"("Numeric"=w388, "Name"=w387) -> ()  [unwired: 9 in, 1 out]
      }
      event "Test Slider": Value Change {
        # "When the test mode slider helper is set, update that\ntree row item's value"
        n259 = event-data() -> ("NewVal"=w394:dbl)  [unwired: 1 in]
        n260 = call <vilib>:"NT Write Number.vi"("Numeric"=w394, "Name"=w395) -> ()  [unwired: 9 in, 1 out]
      }
      event "On/Off": Value Change {
        # "When the test mode on/off helper value is set, update that\ntree row item's value"
        n261 = event-data() -> ("NewVal"=w399:bool)  [unwired: 1 in]
        n262 = Boolean To (0,1)(Boolean=w399) -> (0, 1=w398:i16)
        n263 = call <vilib>:"NT Write Number.vi"("Numeric"=w398, "Name"=w397) -> ()  [unwired: 9 in, 1 out]
      }
      event "Rev/Fwd": Value Change {
        # "When the test mode helper value for relays is set, update that\ntree row item's value"
        n264 = event-data() -> ("NewVal.Forward"=w407:bool, "NewVal.Reverse"=w406:bool)  [unwired: 1 in]
        n265 = Boolean To (0,1)(Boolean=w407) -> (0, 1=w403:i16)
        n266 = Boolean To (0,1)(Boolean=w406) -> (0, 1=w405:i16)
        n267 = Negate(x=w405) -> (-x=w404:i16)
        n268 = Add(x=w403, y=w404) -> (x+y=w402:i16)
        n269 = call <vilib>:"NT Write Number.vi"("Numeric"=w402, "Name"=w401) -> ()  [unwired: 9 in, 1 out]
      }
      event "Test Ring": Value Change {
        # "When a test mode helper value is selected from the ring,\nset the tree item's variable to the string value"
        n270 = event-data() -> ("NewVal"=w411:u16)  [unwired: 1 in]
        n271 = property on="Test Ring" class="Ring (strict)"() -> ("Strings []"=w412:string[])  [unwired: 2 in, 2 out]
        n272 = Index Array(array=w412, index=w411) -> (element=w410:string)
        n273 = call <vilib>:"NT Write String.vi"("String"=w410, "Name"=w409) -> ()  [unwired: 9 in, 1 out]
      }
      event "Rec Mode": Value Change {
        # "Update globals for recording mode and path to read log from.\nClear when logging and let NetworkTables set path for vision to\nuse."
        n274 = event-data() -> ("NewVal"=w423:enum32{"Stop", "Record", "Playback"})  [unwired: 1 in]
        n275 = global write "WPI_DashboardLogging Global.vi" "Logging Filename"(path "") -> ()
        n276 = global write "WPI_DashboardLogging Global.vi" "Recording"(w423) -> ()
        n277 = case shown="\"Playback\"" w423 {
          tunnel: w422 -> [_ w425 w434]
          tunnel: [_ _ w433] -> w420
          tunnel: [_ _ w432] -> _
          tunnel: w418 -> [_ _ w430]
          tunnel: cluster{i32, i32} {-250, 170} -> [_ _ w429]
          tunnel: [_ _ T19 {"Image Size"=TRUE, "Image Type"=TRUE, "Pixel Value"=TRUE, "ROI Information"=TRUE, "Zoom Factor"=FALSE} ("Image Information Shown:All Elements")] -> w416
          tunnel: [_ _ TRUE ("Zoom Factor")] -> w415
          tunnel: w414 -> [_ _ w426]
          frame Default {
          }
          frame "Stop", "Record" {
            # "Place Window too"
            n278 = invoke class="VI" method="FP.Close"(reference=w425) -> (reference out=w424:refnum<vi>)  [unwired: 2 in, 2 out]
            n279 = invoke class="VI" method="Abort VI"(reference=w424) -> ()  [unwired: 2 in, 3 out]
          }
          frame "Playback" {
            n280 = call "Open Playback Panel.vi"("Offset"=w429, "DB VI Ref"=w430, "Playback in"=w434) -> ("Playback out"=w431:refnum<vi>)  [unwired: 8 in]
            n281 = register-events(w431, w426) -> (reference out=w433:refnum<event-registration>, error out=w432:errorcluster)  [unwired: 2 in]
          }
        }
        n282 = property on="Camera Image" class="ImageControl"("Image Information Shown"=w416, "Image Information Visible"=w415) -> ()  [unwired: 2 in, 2 out]
        n283 = call <vilib>:"WPI_DashboardNT Log FieldName Cache.vi"("Operation"=enum16{"Lookup/Add", "Index", "Clear"}."Clear") -> ()  [unwired: 8 in, 3 out]
      }
      event Panel Close {
        w436 = enum32{"Stop", "Record", "Playback"}."Stop" ("Rec Mode")
        # "Playback window has been closed, abort"
        n284 = event-data() -> ()  [unwired: 1 in, 4 out]
        n285 = local write "Rec Mode"(w436) -> ()
        n286 = global write "WPI_DashboardLogging Global.vi" "Recording"(w436) -> ()
      }
      event Panel Close {
        # "Abort playback window and ourself"
        n287 = event-data() -> ()  [unwired: 1 in, 4 out]
        n288 = invoke class="VI" method="FP.Close"(reference=w440) -> (reference out=w439:refnum<vi>)  [unwired: 2 in, 2 out]
        n289 = invoke class="VI" method="Abort VI"(reference=w439) -> (error out=w438:errorcluster)  [unwired: 2 in, 2 out]
        n290 = invoke class="VI" method="Abort VI"(error in=w438) -> ()  [unwired: 2 in, 3 out]
      }
      event User Event {
        n291 = event-data() -> ("IDs"=w447:cluster{"RPC field ID":u16, "Unique ID":u16}, "String"=w446:string)  [unwired: 1 in]
        n292 = Bundle("IDs"=w447, "String"=w446) -> (w445:T8)  [unwired: 1 in]
        n293 = call <vilib>:"Retrieve RPC Response.vi"("RPC Response"=w445) -> ("Output"=w443:string[][])  [unwired: 10 in]
        n294 = Build Array (concatenate)(w441, w443) -> (w442:string[][])
        n295 = local write "Command Params"(w442) -> ()
        n296 = local write "Cmd Status"("" ("Cmd Status")) -> ()
      }
      event "Tree": Double Click {
        n297 = event-data() -> ("PlatMods"=w451:T22, "Tag"=w450:string)  [unwired: 1 in]
        n298 = Unbundle(w451) -> ("Shift"=w449:bool)  [unwired: 4 out]
        n299 = Not(x=w449) -> (.not. x?=w448:bool)
        n300 = call <vilib>:"NT Update Persistence.vi"("Persistence"=w448, "Name"=w450) -> ()  [unwired: 9 in, 1 out]
      }
    }
  }
  n301 = call "IMAQ Create"("Image Name"="Mask", "Image Type"=w3) -> ()  [unwired: 2 in, 3 out]
  n302 = call "IMAQ Create"("Image Name"="Mask2", "Image Type"=w5) -> ("New Image"=w1:T5)  [unwired: 2 in, 2 out]
  n303 = while {
    tunnel: w14 -> [w465]
    tunnel: w13 -> [_]
    tunnel: [w459] -> _
    tunnel: w1 -> [w453]
    i -> [w459]
    stop <- FALSE stop-if-true
    n304 = local read "Rec Mode"() -> (w463:enum32{"Stop", "Record", "Playback"})
    n305 = local read "Robot IP"() -> (w464:string)
    n306 = call <vilib>:"WPI_CameraRead MJPG for Dashboard.vi"("Camera Settings"="Camera Settings Right", "Rec Mode"=w463, "Robot IP"=w464, "Camera Name"="Camera Name Right", "Refnum in"=w465) -> ("Active"=w458:bool, "Refnum out"=w461:T5, "FPS"=w456:dbl, "Bandwidth (Mbps)"=w457:dbl)  [unwired: 3 in]
    n307 = case shown="True" w458 {
      tunnel: w461 -> [w467 w472]
      tunnel: w457 -> [_ _]
      tunnel: w456 -> [_ _]
      tunnel: [w467 w471] -> w455
      tunnel: "LED Color" -> [_ w470]
      tunnel: w453 -> [_ w469]
      frame False {
        n308 = Wait Until Next ms Multiple(millisecond multiple=u32 500) -> ()  [unwired: 1 out]
      }
      frame True {
        n309 = call "BB_Image_Process.vi"("LED Color"=w470, "Mask"=w469, "Input Image"=w472) -> ("Original Image"=w471:T5)  [unwired: 7 in, 1 out]
      }
    }
    "Camera Image Right" <- w455
  }
  n310 = while {
    tunnel: w69 -> [w474]
    i -> [w477]
    stop <- FALSE stop-if-true
    n311 = Wait (ms)(milliseconds to wait=u32 100) -> ()  [unwired: 1 out]
    n312 = case shown="\"Playback\"" "Rec Mode" {
      tunnel: w477 -> [_ _ w492]
      tunnel: [u32 2829099 ("Base Color") u32 11141120 ("Target Color") w481] -> w473
      frame "Stop", Default {
        # "Reset the color, extra updates don't cost much"
      }
      frame "Record" {
      }
      frame "Playback" {
        # "Playback"
        n313 = Quotient & Remainder(x=w492, y=u32 50 ("milliseconds to wait")) -> (x-y*floor(x/y)=w488:u32)  [unwired: 1 out]
        n314 = Divide(x=w488, y=u32 50 ("milliseconds to wait")) -> (x/y=w485:dbl)
        n315 = Multiply(x=6.283185307179586, y=w485) -> (x*y=w490:dbl)
        n316 = Sine(x=w490) -> (sin(x)=w489:dbl)
        n317 = Absolute Value(x=w489) -> (abs(x)=w482:dbl)
        n318 = call "Interpolate RGB Color.vi"("Proportion"=w482, "Target Color"=u32 30976, "Base Color"=u32 2829099) -> ("Result Color"=w481:u32)  [unwired: 8 in]
      }
    }
    n319 = property class="Pane"(reference=w474, "PaneColor"=w473) -> ()  [unwired: 1 in, 2 out]
  }
  n320 = local write "Dashboard Tab"(T3."Drive" ("Dashboard Tab")) -> ()
  n321 = property on="On/Off" class="Bool (strict)"("Visible"=w38) -> ()  [unwired: 2 in, 2 out]
  n322 = property on="Motor" class="Clust (strict)"("Visible"=w38) -> ()  [unwired: 2 in, 2 out]
  n323 = property on="Progress" class="Clust (strict)"("Visible"=w38) -> ()  [unwired: 2 in, 2 out]
  n324 = property on="Test Ring" class="Ring (strict)"("Visible"=w38) -> ()  [unwired: 2 in, 2 out]
  n325 = property on="Rev/Fwd" class="Clust (strict)"("Visible"=w38) -> ()  [unwired: 2 in, 2 out]
  n326 = while {
    tunnel: u16 1741 ("timeout ms (25000)") -> [w494]
    stop <- FALSE stop-if-true
    n327 = TCP Create Listener(10:w494) -> (0:w493:errorcluster, 3:w495:refnum<k5>)  [unwired: 4 in, 1 out]
    n328 = case shown="No Error" w493 {
      selector: w493 -> [w497 _]
      tunnel: w495 -> [w498 _]
      frame No Error {
        n329 = while {
          tunnel: w498 -> [w501]
          tunnel: w497 -> [w500]
          stop <- FALSE stop-if-true
          n330 = TCP Wait On Listener(8:w500, 11:w501) -> (0:w502:errorcluster, 4:w503:refnum<k5>)  [unwired: 2 in, 3 out]
          n331 = local write "TCP"(w503) -> ()
          n332 = case shown="No Error" w502 {
            frame No Error {
            }
            frame Error {
              n333 = Wait (ms)(milliseconds to wait=u32 1000) -> ()  [unwired: 1 out]
            }
          }
        }
      }
      frame Error {
        n334 = Wait (ms)(milliseconds to wait=u32 1000) -> ()  [unwired: 1 out]
      }
    }
  }
  n335 = local write "Command Selection"(u16 0 ("milliseconds to wait")) -> ()
  n336 = local write "Command Params"(string[][] [] ("Command Params")) -> ()
  n337 = global write "WPI_DashboardLogging Global.vi" "Recording"(w63) -> ()
  n338 = local write "Rec Mode"(w63) -> ()
  n339 = call <vilib>:"NT Write String.vi"("String"="Select Auto", "Name"="Auto Selector") -> ()  [unwired: 9 in, 1 out]
